vi "Get TClk Session Reference.vi"(0 "session in":refnum<class "Digitizer Control.lvclass">, 5 "error in (no error)":errorcluster) -> (14 "session out":refnum<class "Digitizer Control.lvclass">, 15 "tclk session reference":refnum<k20>, 16 "fpga reference":refnum<k20>, 19 "error out":errorcluster)   [LabVIEW 2021, in "Digitizer Control.lvclass"]
doc: "Returns the TClk session reference and the FPGA Target reference.\n\nInput:\n\n<B>session in</B>: The device session.\n\nOutputs:\n\n<B>session out</B>: The device session passed on the <B>session in</B> input.\n\n<B>tclk session reference</B>: The TClk session reference.\n\n<B>fpga reference</B>: The FPGA Target reference."
uses:
  Digitizer Control.lvclass
  Digitizer Control.lvclass/Digitizer Control.ctl
  <instrlib>/FlexRIO/API/Host/v1/NI FlexRIO API v1.lvlib
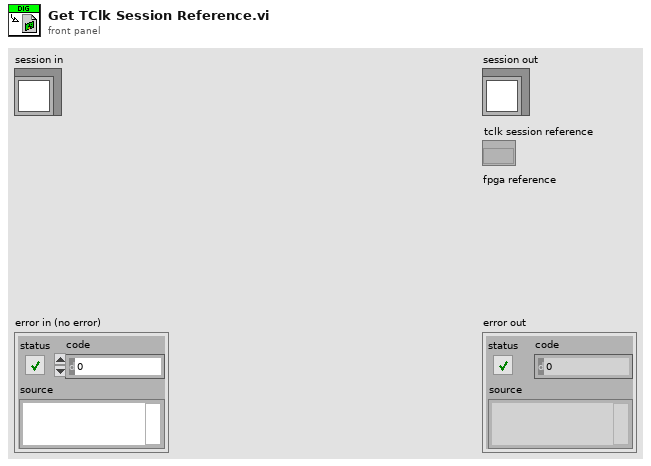
[diagram p1: front panel]
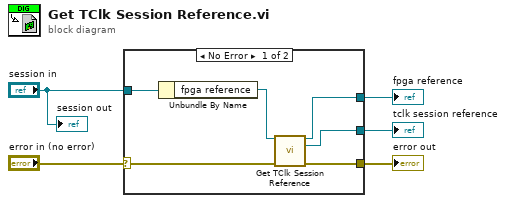
[diagram p0: block diagram]
diagram:
  n1 = case shown="No Error" "error in (no error)" {
    selector: "error in (no error)" -> [w10 w12]
    tunnel: "session in" -> [w11 _]
    tunnel: [w8 _] -> w4
    tunnel: [w7 w12] -> w3
    tunnel: [w6 _] -> w2
    frame No Error {
      n2 = Unbundle By Name(w11) -> ("fpga reference"=w9:refnum<k20>)
      n3 = call <instrlib>:"Get TClk Session Reference.vi"("fpga interface in"=w9, "error in"=w10) -> ("fpga interface out"=w8:refnum<k20>, "tclk session reference"=w6:refnum<k20>, "error out"=w7:errorcluster)  [unwired: 11 in]
    }
    frame Error {
    }
  }
  "error out" <- w3
  "fpga reference" <- w4
  "tclk session reference" <- w2
  "session out" <- "session in"
